vi "FileIO-Append to Text File.vi"(0 "file path":path, 7 "text":string, 11 "error in (no error)":errorcluster) -> (4 "file path out":path, 15 "error out":errorcluster)   [LabVIEW 2020]
doc: "Appends text to the end of a file. Creates the file if it doesn't exist."
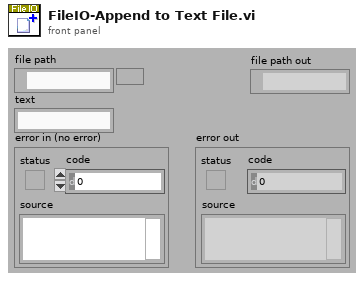
[diagram p1: front panel]
types:
  T1 = enum16{"open", "replace", "create", "open or create", "replace or create", "replace or create with confirmation"}
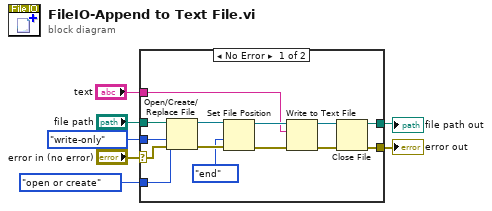
[diagram p0: block diagram]
diagram:
  n1 = case shown="No Error" "error in (no error)" {
    selector: "error in (no error)" -> [w8 w22]
    tunnel: "file path" -> [w21 w23]
    tunnel: enum16{"read/write", "read-only", "write-only"}."write-only" ("access (0:read/write)") -> [w20 _]
    tunnel: "text" -> [w14 _]
    tunnel: [w11 w22] -> w4
    tunnel: [w10 w23] -> w3
    tunnel: T1."open or create" ("operation (0:open)") -> [w9 _]
    frame No Error {
      n2 = Open/Create/Replace File(file path (use dialog)=w21, error in=w8, operation (0:open)=w9, access (0:read/write)=w20) -> (refnum out=w18:refnum<file>, error out=w19:errorcluster)  [unwired: 2 in, 1 out]
      n3 = Set File Position(refnum=w18, from (0:start)=enum16{"start", "end", "current"}."end", error in=w19) -> (refnum out=w15:refnum<file>, error out=w16:errorcluster)  [unwired: 1 in]
      n4 = Write to Text File(file (use dialog)=w15, text=w14, error in=w16) -> (refnum out=w12:refnum<file>, error out=w13:errorcluster)  [unwired: 1 in, 1 out]
      n5 = Close File(refnum=w12, error in=w13) -> (path=w10:path, error out=w11:errorcluster)
    }
    frame Error {
    }
  }
  "error out" <- w4
  "file path out" <- w3
